vi "Parse Error Messages.vi"(8 "error in":errorcluster, 11 "Node in":refnum<k20>) -> (0 "error out":errorcluster, 2 "Errors":T1(array[cluster]), 3 "Node out":refnum<k20>)   [LabVIEW 2024, in "Parser.lvlib"]
uses:
  Parser.lvlib
  <vilib>/xml/Close Reference(Node).vi
  <resource>/objmgr/DOMUserDefRef.rc
  <vilib>/xml/NI_XML.lvlib
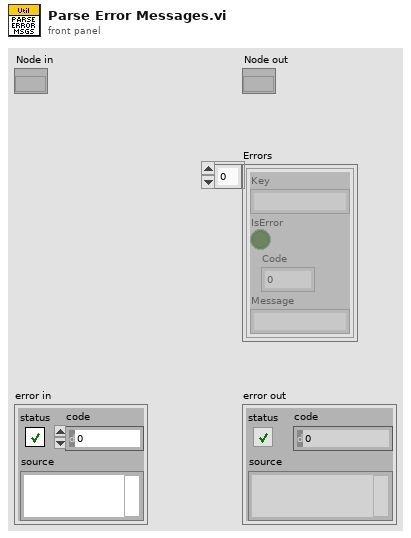
[diagram p1: front panel]
types:
  T1 = cluster{"Key":string, "IsError":bool, "Code":u32, "Message":string}[]
  T2 = cluster{"Key":string, "IsError":bool, "Code":u32, "Message":string}
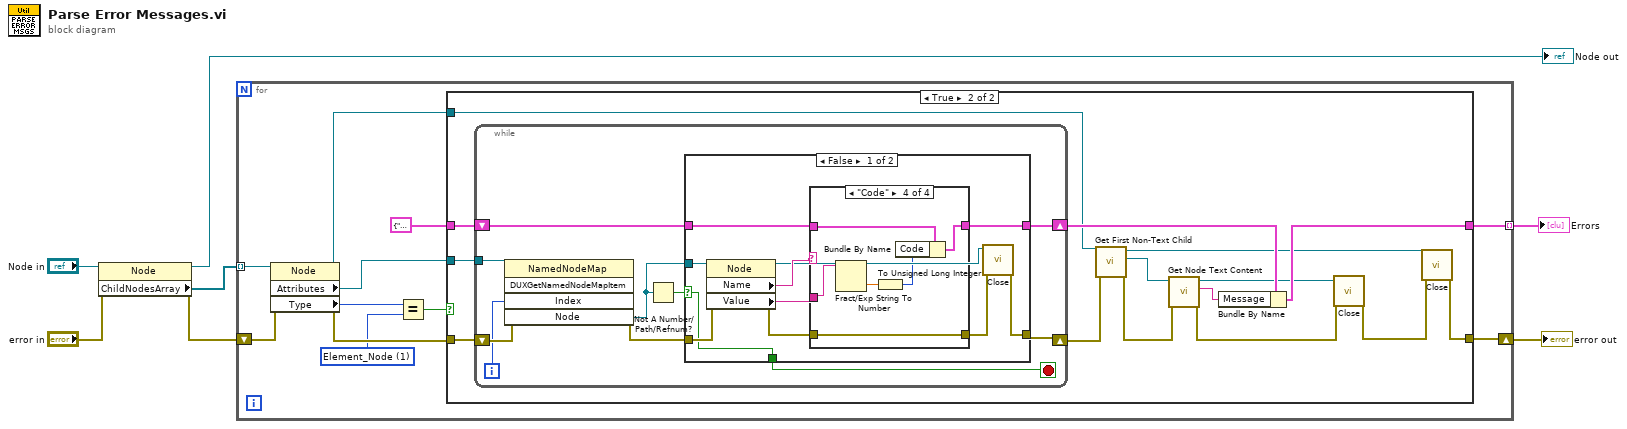
[diagram p0: block diagram]
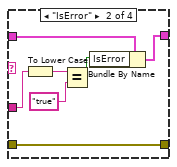
[diagram p4: hidden frame]
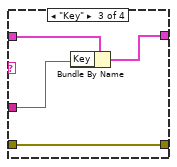
[diagram p5: hidden frame]
diagram:
  n1 = property class="Node"(reference="Node in", error in="error in") -> (reference out=→"Node out":refnum<k20>, error out=w6:errorcluster, "ChildNodesArray"=w2:refnum<k20>[])
  n2 = for {
    tunnel: w2 -> [w14] mode=indexing
    tunnel: [w12] -> w3 mode=indexing
    shift-right: [w16] -> w5
    shift-left: w6 -> [w17]
    w10 = 1 items=["Element_Node"=1, "Attribute_Node"=2, "Text_Node"=3, "CDATASection_Node"=4, "EntityReference_Node"=5, "Entity_Node"=6, "ProcessingInstruction_Node"=7, "Comment_Node"=8, "Document_Node"=9, "DocumentType_Node"=10, "DocumentFragment_Node"=11, "Notation_Node"=12] ("Node Type")
    n3 = property on="Property Node" class="Node"(reference=w14, error in=w17) -> (reference out=w9:refnum<k20>, error out=w18:errorcluster, "Attributes"=w15:refnum<k20>, "Type"=w11:i32)
    n4 = Equal?(x=w11, y=w10) -> (x = y?=w8:bool)
    n5 = case shown="True" w8 {
      tunnel: w18 -> [w20 w35]
      tunnel: [w20 w32] -> w16
      tunnel: w15 -> [_ w29]
      tunnel: T2 {"Key"="", "IsError"=FALSE, "Code"=0, "Message"=""} ("Error") -> [w19 w27]
      tunnel: [w19 w26] -> w12
      tunnel: w9 -> [_ w21]
      frame False {
      }
      frame True {
        n6 = while {
          tunnel: w29 -> [w42]
          shift-right: [w43] -> w34
          shift-left: w35 -> [w45]
          shift-right: [w36] -> w28
          shift-left: w27 -> [w37]
          i -> [w41]
          stop <- w38 stop-if-true
          n7 = invoke on="Invoke Node" class="NamedNodeMap" method="DUXGetNamedNodeMapItem"(reference=w42, error in=w45, "Index"=w41) -> (error out=w44:errorcluster, "Node"=w40:refnum<k20>)  [unwired: 2 in, 3 out]
          n8 = Not A Number/Path/Refnum?(number/path/refnum=w40) -> (NaN/Path/Refnum?=w39:bool)
          n9 = case shown="False" w39 {
            selector: w39 -> [w46 w77]
            tunnel: w44 -> [w56 w78]
            tunnel: [w53 w78] -> w43
            tunnel: w40 -> [w52 _]
            tunnel: [w46 w77] -> w38
            tunnel: w37 -> [w50 w76]
            tunnel: [w48 w76] -> w36
            frame False {
              n10 = property on="Property Node" class="Node"(reference=w52, error in=w56) -> (reference out=w47:refnum<k20>, error out=w55:errorcluster, "Name"=w51:string, "Value"=w49:string)
              n11 = case shown="\"Code\"" w51 {
                tunnel: w50 -> [w57 w64 w68 w74]
                tunnel: w49 -> [_ w62 w67 w72]
                tunnel: [w57 w63 w66 w73] -> w48
                tunnel: w55 -> [w58 w65 w69 w75]
                tunnel: [w58 w65 w69 w75] -> w54
                frame "-1", Default {
                }
                frame "IsError" {
                  n12 = To Lower Case(string=w62) -> (all lower case string=w61:string)
                  n13 = Equal?(x=w61, y="true") -> (x = y?=w59:bool)
                  n14 = Bundle By Name(cluster=w64, "IsError"=w59) -> (w63:T2)
                }
                frame "Key" {
                  n15 = Bundle By Name(cluster=w68, "Key"=w67) -> (w66:T2)
                }
                frame "Code" {
                  n16 = Fract/Exp String To Number(string=w72) -> (number=w71:dbl)  [unwired: 3 in, 1 out]
                  n17 = To Unsigned Long Integer(number=w71) -> (unsigned 32bit integer=w70:u32)
                  n18 = Bundle By Name(cluster=w74, "Code"=w70) -> (w73:T2)
                }
              }
              n19 = call-poly <vilib>:"Close.vi"("error in (no error)"=w54, "node"=w47) -> ("error out"=w53:errorcluster)  [unwired: 7 in]
            }
            frame True {
            }
          }
        }
        n20 = call <vilib>:"Get First Non-Text Child.vi"("error in (no error)"=w34, "node in"=w21) -> ("error out"=w30:errorcluster, "child node"=w23:refnum<k20>, "node out"=w22:refnum<k20>)  [unwired: 6 in, 1 out]
        n21 = call <vilib>:"Get Node Text Content.vi"("error in (no error)"=w30, "node in"=w23) -> ("error out"=w31:errorcluster, "node text"=w24:string, "node out"=w25:refnum<k20>)  [unwired: 7 in]
        n22 = Bundle By Name(cluster=w28, "Message"=w24) -> (w26:T2)
        n23 = call-poly <vilib>:"Close.vi"("error in (no error)"=w31, "node"=w25) -> ("error out"=w33:errorcluster)  [unwired: 7 in]
        n24 = call-poly <vilib>:"Close.vi"("error in (no error)"=w33, "node"=w22) -> ("error out"=w32:errorcluster)  [unwired: 7 in]
      }
    }
  }
  "Errors" <- w3
  "error out" <- w5
